vi "Vision Processing.vi"(4 "error in (no error)":errorcluster, 7 "Image Size":T2=enum."320x240") -> ()   [LabVIEW 2015]
doc: "This VI runs in parallel to other tasks. It gets images from the camera, processes them for color or shape and use that information to affect robot behavior."
uses:
  <vilib>/Rock Robotics/WPI/Camera/WPI_CameraImageSize.ctl
  Program Files (x86)/National Instruments/LabVIEW 2015/examples/FRC/roboRIO/Vision/2016 Vision Example/Vision Support Code/Camera Types.ctl
  <vilib>/Rock Robotics/WPI/Camera/WPI_CameraWhite Balance Values.ctl
  <vilib>/Rock Robotics/WPI/Camera/WPI_CameraExposure Values.ctl
  <vilib>/Rock Robotics/WPI/Camera/WPI_CameraFrameRate.ctl
  Robot Global Data.vi
  Globales/Vision Scores Global.vi
  <vilib>/vision/NI_Vision_Development_Module.lvlib
panel:
  in  "Camera Type":T1=enum."1011"
  out "ms to process":u32
  in  "LED Color":T3={"Hue"={23.67058792990901, 48.923317529462665}, "Sat"={66.78571428571429, 255.0}, "Val"={48.571428571428584, 255.0}} {"Hue" scale=0.0..255.0 scale format="%#_3g"}
  out "Qualified Particles":i32
  in  "Score Threshold":dbl=75.0
  in  "Aspect Fudge Factor":dbl=1.0
  in  "Min Score Threshold":i32=75
  in  "Emphasize Limit Tests":bool=TRUE
  out "Masked":T4(plugin-control)
  in  "Display Mask":bool=TRUE
  out "Original Image":T4(plugin-control)
  in  "Display Original":bool=TRUE
  out "Sorted Particle Scores":T5(array[cluster]) {"Moment Factor" format="%#_3g"; "Aspect Ratio" format="%#_3g"; "Area to CH" format="%#_3g"; "X" format="%#_3g"; "Y" format="%#_3g"}
  out "Highest Avg Score":dbl
  out "Detected Targets":T6(array[cluster]) {"Normalized Rect"."Numeric 5" format="%#_2g"; "Normalized Rect"."Numeric 3" format="%#_2g"; "Normalized Rect"."Numeric 2" format="%#_2g"; "Normalized Rect"."Numeric" format="%#_2g"}
  out "fps":dbl
  # "Density Profile"
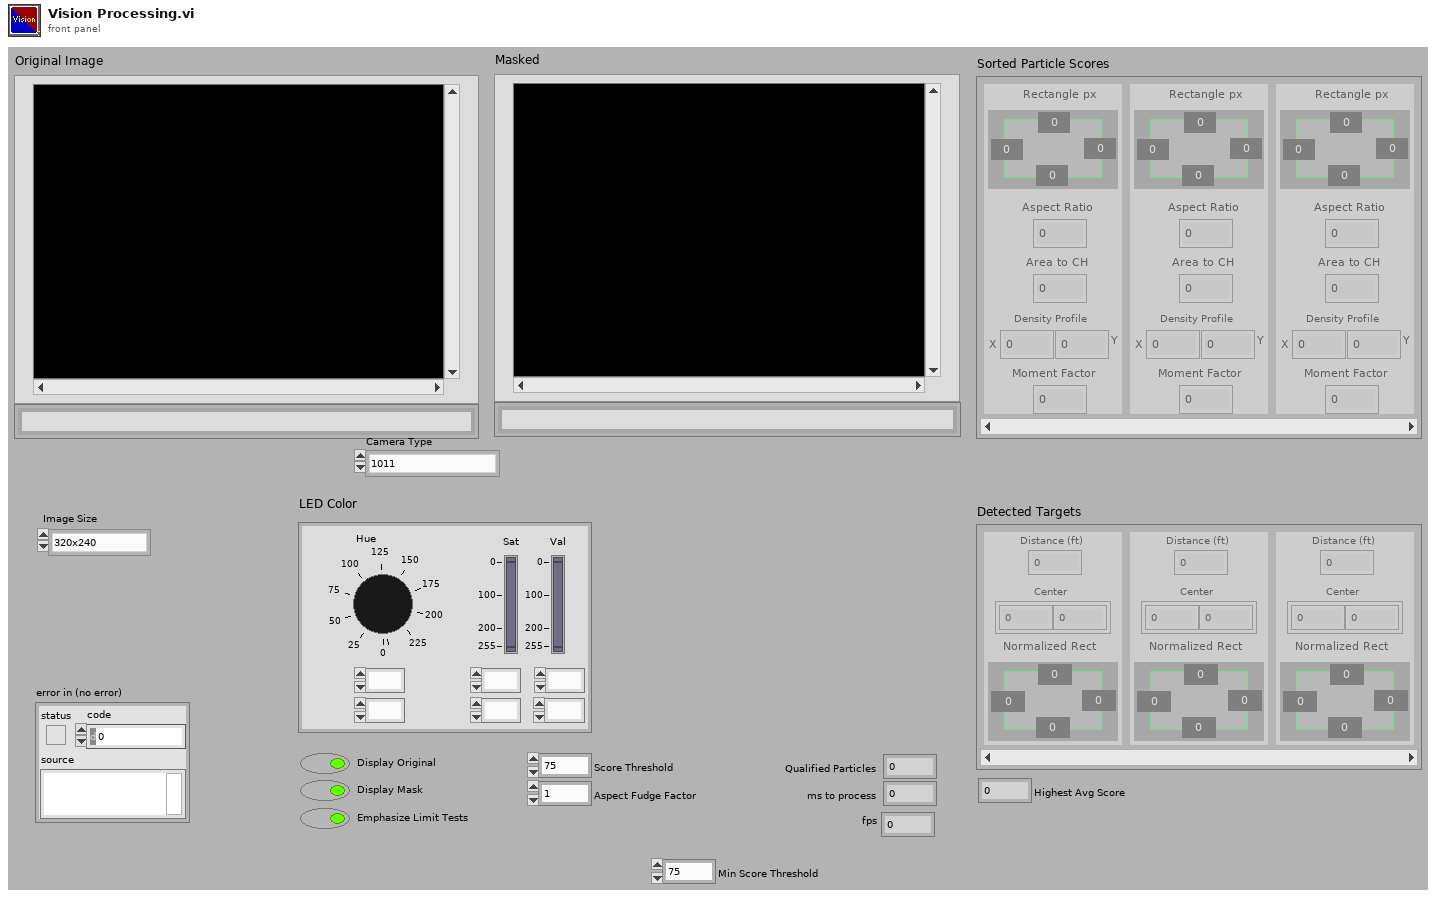
[diagram p1: front panel]
types:
  T1 = typedef "Camera Types.ctl" = enum16{"206", "1011", "1013", "MS HD3000 square", "MS HD3000 640x480"}
  T2 = typedef "WPI_CameraImageSize.ctl" = enum16{"640x480", "320x240", "160x120", "Custom"}
  T3 = cluster{"Hue":cluster{dbl, dbl}, "Sat":cluster{dbl, dbl}, "Val":cluster{dbl, dbl}}
  T4 = typedef "IMAQ Image.ctl" = refnum<image>
  T5 = cluster{"Rectangle px":cluster{"Numeric":dbl, "Numeric 2":dbl, "Numeric 3":dbl, "Numeric 5":dbl}, "Aspect Ratio":dbl, "Area to CH":dbl, "X":dbl, "Y":dbl, "Moment Factor":dbl}[]
  T6 = cluster{"Distance (ft)":dbl, "Center":cluster{dbl, dbl}, "Normalized Rect":cluster{"Numeric":dbl, "Numeric 2":dbl, "Numeric 3":dbl, "Numeric 5":dbl}}[]
  T7 = typedef "WPI_CameraFrameRate.ctl" = u32
  T8 = typedef "WPI_CameraExposure Values.ctl" = enum16{"Auto", "Flicker-free 50 Hz", "Flicker-free 60 Hz", "Hold current", "Custom"}
  T9 = typedef "WPI_CameraWhite Balance Values.ctl" = enum16{"Auto", "Fixed indoor", "Fixed outdoor 1", "Fixed outdoor 2", "Fixed fluorescent 1", "Fixed fluorescent 2", "Hold current", "Custom"}
  T10 = typedef "Particle Parameters" = i32
  T11 = typedef "Image Type" = u32
  T12 = typedef "WPI_CameraDevRef.ctl" = cluster{"Camera Address":string, "CameraStatus":errorcluster}
  T13 = cluster{"Bounding box":cluster{"left":dbl, "top":dbl, "right":dbl, "bottom":dbl}, "Aspect Ratio":dbl, "Area to CH":dbl, "X Mask":dbl, "Y Mask":dbl, "Moment":dbl}[]
  T14 = cluster{"Rectangle":cluster{"Numeric":dbl, "Numeric 2":dbl, "Numeric 3":dbl, "Numeric 5":dbl}, "L":dbl, "Area to CH":dbl, "X":dbl, "Y":dbl, "Moment Factor":dbl}[]
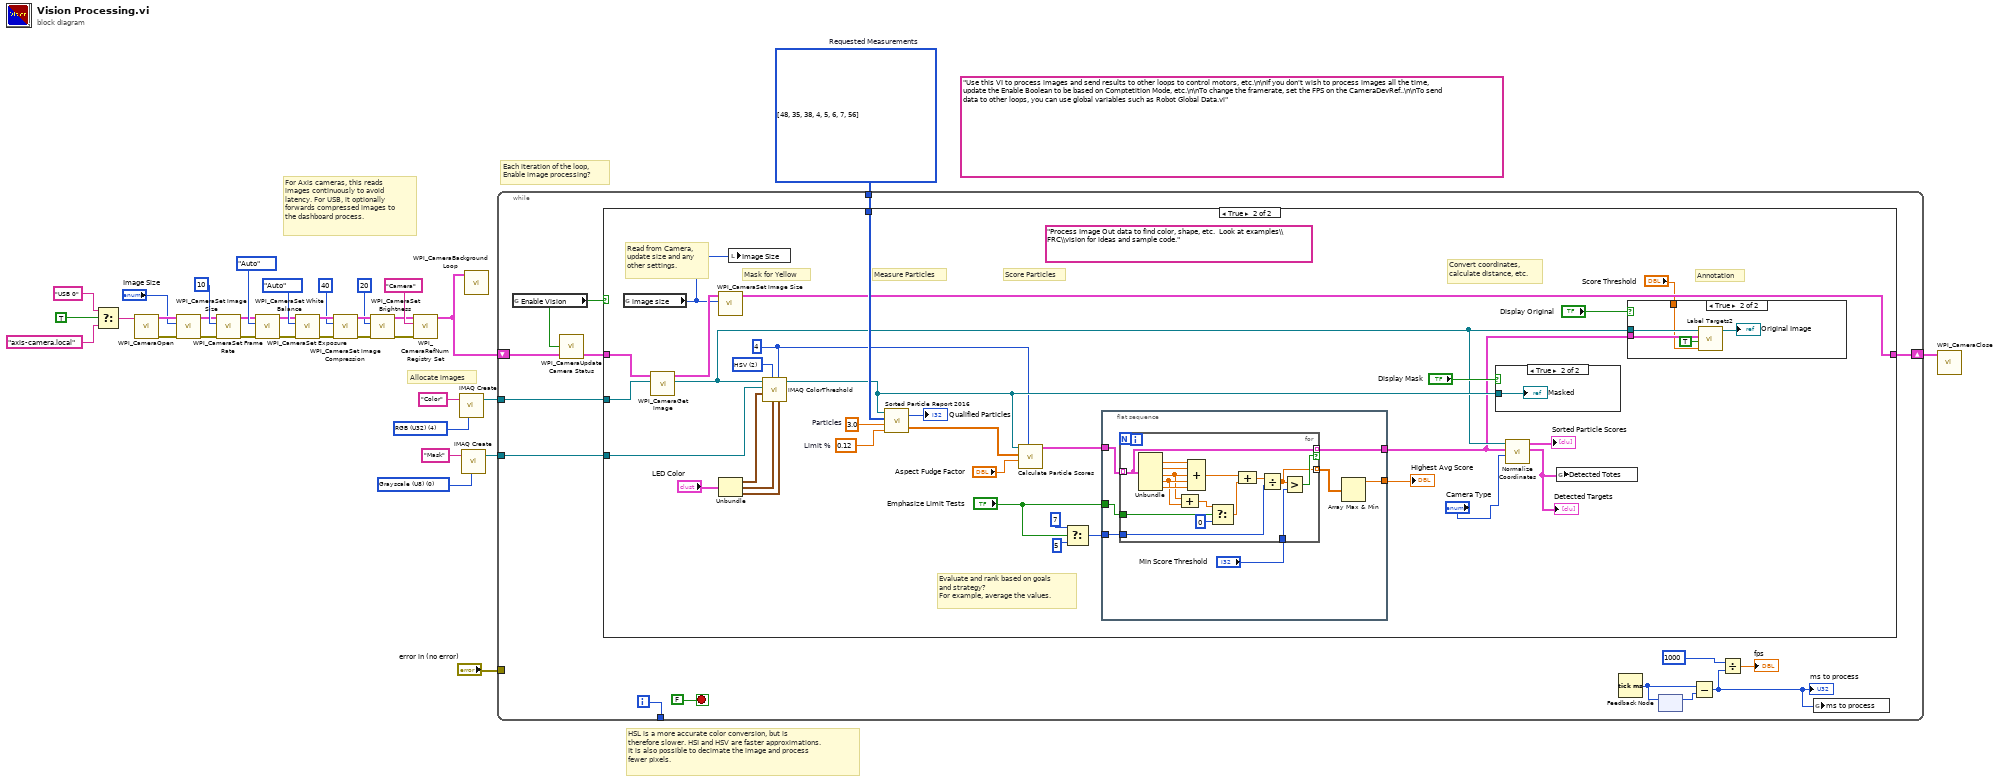
[diagram p0: block diagram]
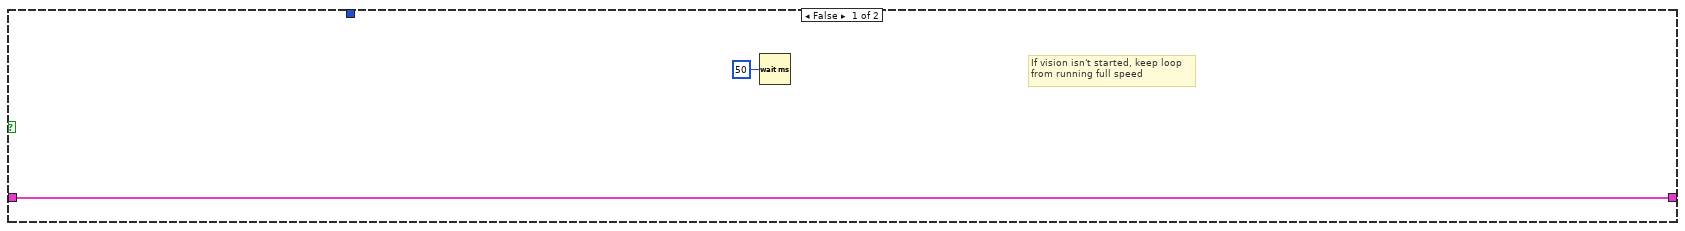
[diagram p2: hidden frame]
diagram:
  (unwired) "Use this VI to process images and send results to other loops to control motors, etc.\n\nIf you don't wish to process images all the time, update the Enable Boolean to be based on Comptetition Mode, etc.\n\nTo change the framerate, set the FPS on the CameraDevRef..\n\nTo send data to other loops, you can use global variables such as Robot Global Data.vi"
  w29 = T10[] [48, 35, 38, 4, 5, 6, 7, 56] items=["Center of Mass X", "Center of Mass Y", "First Pixel X", "First Pixel Y", "Bounding Rect Left", "Bounding Rect Top", "Bounding Rect Right", "Bounding Rect Bottom", "Max Feret Diameter Start X", "Max Feret Diameter Start Y", "Max Feret Diameter End X", "Max Feret Diameter End Y", "Max Horiz. Segment Length Left", "Max Horiz. Segment Length Right", "Max Horiz. Segment Length Row", "-", "Bounding Rect Width", "Bounding Rect Height", "Bounding Rect Diagonal", "Perimeter", "Convex Hull Perimeter", "Holes' Perimeter", "Max Feret Diameter", "Equivalent Ellipse Major Axis", "Equivalent Ellipse Minor Axis", "Equivalent Ellipse Minor Axis (Feret)", "Equivalent Rect Long Side", "Equivalent Rect Short Side", "Equivalent Rect Diagonal", "Equivalent Rect Short Side (Feret)", "Average Horiz. Segment Length", "Average Vert. Segment Length", "Hydraulic Radius", "Waddel Disk Diameter", "-", "Area", "Holes' Area", "Particle & Holes' Area", "Convex Hull Area", "Image Area", "-", "Number of Holes", "Number of Horiz. Segments", "Number of Vert. Segments", "-", "Orientation", "Max Feret Diameter Orientation", "-", "% Area/Image Area", "% Area/(Particle & Holes' Area)", "Ratio of Equivalent Ellipse Axes", "Ratio of Equivalent Rect Sides", "-", "Elongation Factor", "Compactness Factor", "Heywood Circularity Factor", "Type Factor", "-", "Sum X", "Sum Y", "Sum XX", "Sum XY", "Sum YY", "Sum XXX", "Sum XXY", "Sum XYY", "Sum YYY", "-", "Moment of Inertia XX", "Moment of Inertia XY", "Moment of Inertia YY", "Moment of Inertia XXX", "Moment of Inertia XXY", "Moment of Inertia XYY", "Moment of Inertia YYY", "Norm. Moment of Inertia XX", "Norm. Moment of Inertia XY", "Norm. Moment of Inertia YY", "Norm. Moment of Inertia XXX", "Norm. Moment of Inertia XXY", "Norm. Moment of Inertia XYY", "Norm. Moment of Inertia YYY", "Hu Moment 1", "Hu Moment 2", "Hu Moment 3", "Hu Moment 4", "Hu Moment 5", "Hu Moment 6", "Hu Moment 7"]  # Requested Measurements
  w32 = T11 0 items=["Grayscale (U8)", "Grayscale (I16)", "Grayscale (SGL)", "Complex (CSG)", "RGB (U32)", "HSL (U32)", "RGB (U64)", "Grayscale (U16)"] ("Image Type")
  w34 = T11 4 items=["Grayscale (U8)", "Grayscale (I16)", "Grayscale (SGL)", "Complex (CSG)", "RGB (U32)", "HSL (U32)", "RGB (U64)", "Grayscale (U16)"] ("Image Type")
  # "Each iteration of the loop,\nEnable image processing?"
  # "HSL is a more accurate color conversion, but is\ntherefore slower. HSI and HSV are faster approximations.\nIt is also possible to decimate the image and process\nfewer pixels."
  # "For Axis cameras, this reads\nimages continuously to avoid\nlatency. For USB, it optionally\nforwards compressed images to\nthe dashboard process."
  # "Allocate images"
  n1 = Select(t="USB 0" ("format string"), s=TRUE ("dot notation? (F)"), f="axis-camera.local" ("format string")) -> (s? t:f=w28:string)
  n2 = call <vilib>:"WPI_CameraOpen.vi"("Camera Address"=w28) -> ("error out"=w16:errorcluster, "CameraDevRef"=w15:T12)  [unwired: 1 in, 8 out]
  n3 = call <vilib>:"WPI_CameraSet Image Size.vi"("error in (no error)"=w16, "Image Size"="Image Size", "CameraDevRef"=w15) -> ("error out"=w17:errorcluster, "CameraDevRef Out"=w14:T12)  [unwired: 1 in, 6 out]
  n4 = call <vilib>:"WPI_CameraSet Frame Rate.vi"("error in (no error)"=w17, "Frame Rate (fps)"=T7 10, "CameraDevRef"=w14) -> ("error out"=w18:errorcluster, "CameraDevRef Out"=w12:T12)  [unwired: 7 out]
  n5 = call <vilib>:"WPI_CameraSet White Balance.vi"("error in (no error)"=w18, "White Balance"=WPI_CameraWhite_Balance_Values."Auto", "CameraDevRef"=w12) -> ("error out"=w19:errorcluster, "CameraDevRef Out"=w13:T12)  [unwired: 1 in, 6 out]
  n6 = call <vilib>:"WPI_CameraSet Exposure.vi"("error in (no error)"=w19, "Exposure"=WPI_CameraExposure_Values."Auto", "CameraDevRef"=w13) -> ("error out"=w20:errorcluster, "CameraDevRef Out"=w10:T12)  [unwired: 1 in, 6 out]
  n7 = call <vilib>:"WPI_CameraSet Image Compression.vi"("error in (no error)"=w20, "Compression"=40, "CameraDevRef"=w10) -> ("error out"=w21:errorcluster, "CameraDevRef Out"=w11:T12)  [unwired: 7 out]
  n8 = call <vilib>:"WPI_CameraSet Brightness.vi"("error in (no error)"=w21, "Brightness"=20, "CameraDevRef"=w11) -> ("error out"=w22:errorcluster, "CameraDevRef Out"=w1:T12)  [unwired: 7 out]
  n9 = call <vilib>:"WPI_CameraRefNum Registry Set.vi"("error in (no error)"=w22, "refnum name"="Camera", "CameraDevRef"=w1) -> ("CameraDevRef"=w6:T12)  [unwired: 1 in, 7 out]
  n10 = call "IMAQ Create"("Image Name"="Color", "Image Type"=w34) -> ("New Image"=w33:T4)  [unwired: 2 in, 2 out]
  n11 = call "IMAQ Create"("Image Name"="Mask", "Image Type"=w32) -> ("New Image"=w30:T4)  [unwired: 2 in, 2 out]
  n12 = call <vilib>:"WPI_CameraBackground Loop.vi"("CameraDevRef"=w6) -> ()  [unwired: 11 in]
  n13 = while {
    tunnel: w33 -> [w44]
    tunnel: w30 -> [w48]
    tunnel: w29 -> [w47]
    tunnel: "error in (no error)" -> [_]
    tunnel: [w43] -> _
    shift-right: [w39] -> w2
    shift-left: w6 -> [w41]
    i -> [w43]
    stop <- FALSE stop-if-true
    n14 = global read "Robot Global Data.vi" "Enable Vision"() -> (w42:bool)
    n15 = call <vilib>:"WPI_CameraUpdate Camera Status.vi"("CameraDevRef In"=w41, "Enable Vision"=w42) -> ("CameraDevRef Out"=w40:T12)  [unwired: 3 in]
    n16 = case shown="True" w42 {
      tunnel: w48 -> [_ w84]
      tunnel: w47 -> [_ w79]
      tunnel: w40 -> [w50 w75]
      tunnel: w44 -> [_ w74]
      tunnel: [w50 w72] -> w39
      frame False {
        # "If vision isn't started, keep loop\nfrom running full speed"
        n17 = Wait (ms)(milliseconds to wait=u32 50) -> ()  [unwired: 1 out]
      }
      frame True {
        w56 = 4 ("Replace Value")
        w69 = u16 2 items=["RGB", "HSL", "HSV", "HSI"] ("Color Mode")
        (unwired) "Process Image Out data to find color, shape, etc.  Look at examples\\FRC\\vision for ideas and sample code."
        w76 = 0.12  # Limit %
        w78 = 3.0  # Particles
        # "Evaluate and rank based on goals\nand strategy?\nFor example, average the values."
        # "Read from Camera,\nupdate size and any\nother settings."
        # "Measure Particles"
        # "Convert coordinates,\ncalculate distance, etc."
        # "Annotation"
        # "Score Particles"
        # "Mask for Yellow"
        n18 = global read "Robot Global Data.vi" "image size"() -> (w54:T2)
        n19 = call <vilib>:"WPI_CameraGet Image.vi"("Image"=w74, "CameraDevRef"=w75) -> ("Image Out"=w59:T4, "CameraDevRef Out"=w73:T12)  [unwired: 7 in, 1 out]
        n20 = call <vilib>:"WPI_CameraSet Image Size.vi"("Image Size"=w54, "CameraDevRef"=w73) -> ("CameraDevRef Out"=w72:T12)  [unwired: 2 in, 7 out]
        n21 = Unbundle("LED Color") -> ("Hue"=w83:cluster{dbl, dbl}, "Sat"=w82:cluster{dbl, dbl}, "Val"=w81:cluster{dbl, dbl})
        n22 = local write "Image Size"(w54) -> ()
        n23 = call "IMAQ ColorThreshold"("Blue or Luma or Val or Inten Range"=w81, "Replace Value"=w56, "Green or Sat Range"=w82, "Color Mode"=w69, "Red or Hue Range"=w83, "Image Dst"=w84, "Image Src"=w59) -> ("Image Dst Out"=w68:T4)  [unwired: 3 in, 1 out]
        n24 = call "Sorted Particle Report 2016.vi"("Min Area Size %"=w76, "Particle Count Limit"=w78, "Pixel Measurements"=w79, "Image in"=w68) -> ("Sorted Data"=w67:dbl[][], "Particles"=→"Qualified Particles":i32)
        n25 = call "Calculate Particle Scores.vi"("Pixel Value"=w56, "Aspect Fudge Factor"="Aspect Fudge Factor", "Sorted Data"=w67, "Image in"=w68) -> ("Scores"=w65:T13)  [unwired: 7 in]
        n26 = Select(t=7, s="Emphasize Limit Tests", f=5) -> (s? t:f=w62:i32)
        n27 = flat-sequence {
          tunnel: w65 -> [w96]
          tunnel: w62 -> [w94]
          tunnel: [w97] -> w61
          tunnel: [w91] -> w58
          tunnel: "Emphasize Limit Tests" -> [w95]
          frame #0 {
            n28 = for {
              tunnel: w96 -> [w111] mode=indexing
              tunnel: [w111] -> w91 mode=indexing if=w110
              tunnel: [w109] -> w92 mode=indexing
              tunnel: w94 -> [w108]
              tunnel: "Min Score Threshold" -> [w107]
              tunnel: w95 -> [w100]
              n29 = Unbundle(w111) -> ("Aspect Ratio"=w113:dbl, "Area to CH"=w112:dbl, "X Mask"=w102:dbl, "Y Mask"=w103:dbl, "Moment"=w104:dbl)  [unwired: 1 out]
              n30 = Compound Arithmetic op=ADD(w102, w103) -> (w101:dbl)
              n31 = Compound Arithmetic op=ADD(w113, w112, w102, w103, w104) -> (w106:dbl)
              n32 = Select(t=w101, s=w100, f=0) -> (s? t:f=w99:dbl)
              n33 = Compound Arithmetic op=ADD(w106, w99) -> (w105:dbl)
              n34 = Divide(x=w105, y=w108) -> (x/y=w109:dbl)
              n35 = Greater?(x=w109, y=w107) -> (0:w110:bool)
            }
            n36 = Array Max & Min(array=w92) -> (max value=w97:dbl)  [unwired: 3 out]
          }
        }
        n37 = case shown="True" "Display Mask" {
          tunnel: w68 -> [_ w90]
          frame False {
          }
          frame True {
            "Masked" <- w90
          }
        }
        n38 = call "Normalize Coordinates.vi"("Camera Type"="Camera Type", "Targets"=w58, "Image in"=w59) -> ("Found Targets"=w55:T6, "Sorted Scores"=→"Sorted Particle Scores":T14)  [unwired: 7 in]
        "Detected Targets" <- w55
        n39 = global write "Vision Scores Global.vi" "Detected Totes"(w55) -> ()
        n40 = case shown="True" "Display Original" {
          tunnel: w59 -> [_ w89]
          tunnel: w58 -> [_ w87]
          tunnel: "Score Threshold" -> [_ w86]
          frame False {
          }
          frame True {
            n41 = call "Label Targets2.vi"("Score Threshold"=w86, "Annotate"=TRUE, "Targets"=w87, "Image in"=w89) -> ("Image out"=→"Original Image":T4)  [unwired: 7 in]
          }
        }
        "Highest Avg Score" <- w61
      }
    }
    n42 = Tick Count (ms)() -> (millisecond timer value=w45:u32)
    n43 = feedback-in #1(w45) -> ()
    n44 = feedback #1() -> (w46:u32)  [unwired: 1 in]
    n45 = Subtract(x=w45, y=w46) -> (x-y=w38:u32)
    "ms to process" <- w38
    n46 = Divide(x=1000 ("Brightness"), y=w38) -> (x/y=→"fps":dbl)
    n47 = global write "Vision Scores Global.vi" "ms to process"(w38) -> ()
  }
  n48 = call <vilib>:"WPI_CameraClose.vi"("CameraDevRef"=w2) -> ()  [unwired: 1 in, 10 out]
